vi "svfa_Process Frequency Response Subset.vi"(0 "Windowed signal [X]":waveform(dbl)={"t0"=timestamp(0 s since 1904-01-01), "dt"=1.953125e-05, "Y"=[]}, 1 "Windowed signal [Y]":waveform(dbl)={"t0"=timestamp(0 s since 1904-01-01), "dt"=1.953125e-05, "Y"=[]}, 2 "window (includes Force_Exp)":T9(ring), 3 "force/exp settings":T8={"force window [%]"=50.0, "exponential window [%]"=10.0} {"exponential window [%]" min=0.0 max=100.0 format="%.2f"; "force window [%]" min=0.0 max=100.0 format="%.2f"}, 4 "averaging parameters":T12={"averaging mode"=enum."No averaging", "weighting mode"=enum."Linear", "number of averages"=10, "linear mode"=enum."Auto restart"}, 5 "error in (no error)":errorcluster, 6 "Spectrum Settings":T10 {"stop frequency" format="%.2f"; "start frequency" format="%.2f"}, 7 "processing control":T7(ring), 9 "FRF mode":enum16{"H1", "H2", "H3"}(ring)) -> (12 "averages completed":dbl format="%.2f", 13 "processing control":T7(ring), 14 "complex frequency response":T11={"f0"=0.0, "df"=1.0, "complex spectrum"=[]} {"complex spectrum" format="%.2f"; "df" format="%.2f"; "f0" format="%.2f"}, 16 "Coherence":cluster{"f0":dbl, "df":dbl, "Spectrum":dbl[]} {"Spectrum" format="%.2f"; "df" format="%.2f"; "f0" format="%.2f"}, 17 "averaging done":bool, 18 "spectrum info":T1={"channel name"="", "description"="", "x-axis units"=0, "spectral info"={"spectrum type"=enum."Power [Magnitude^2]", "linear/dB"=enum."linear", "window"=0, "window size"=0, "FFT size"=0}, "engineering units"=1, "custom label"="", "dB reference [EU]"=0.0, "peak units"=enum."rms", "weighting filter"=0, "spectral density?"=FALSE, "unit label"="", "spectrum skewed?"=FALSE, "complimentary spectrum units"=enum."none"} {"x-axis units" items=["Time (s)"=0, "Frequency-CB (Hz)"=1, "Frequency-CPB (Hz)"=1248, "Frequency-Arbitrary (Hz)"=2357, "Quefrency (s)"=2, "Revolutions (rev)"=3, "Order"=4, "Speed (RPM)"=11, "Speed (rad/s)"=21, "Index"=65535]; "weighting filter" items=["Linear", "A-weighting", "B-weighting", "C-weighting", "ITU-R 468-4", "Dolby", "CCITT", "C-message", "Wb", "Wc", "Wd", "We", "Wf", "Wh", "Wj", "Wk", "Wm", "AES17 20 kHz lowpass", "AES17 40 kHz lowpass", "AES17 20 kHz highpass", "AES17 40 kHz highpass"]; "dB reference [EU]" format="%.2f"; "engineering units" items=["custom..."=0, "V"=1, "A"=21, "C"=30, "pC"=31, "s"=32, "-"=29, "Pa"=2, "N"=20, "g"=3, "m/s^2"=4, "m/s"=5, "m"=6, "mm/s"=12, "mm"=13, "micron/s"=14, "micron"=15, "in/s^2"=7, "in/s"=8, "in"=9, "mil/s"=10, "mil"=11, "rad/s^2"=16, "rad/s"=17, "rad"=18, "deg/s^2"=26, "deg/s"=27, "deg"=28, "RPM"=22, "cycle/s^2"=23, "Hz"=24, "cycle"=25, "strain"=19]; "spectral info"."window" items=["None "=0, "Hanning"=1, "Hamming"=2, "Blackman-Harris"=3, "Exact Blackman"=4, "Blackman"=5, "Flat Top"=6, "4 Term B-Harris "=7, "7 Term B-Harris"=8, "Low Sidelobe"=9, "Force - Exponential"=10, "Gaussian"=62]}, 19 "error out":errorcluster)   [LabVIEW 2017]
uses:
  <vilib>/addons/_NISVFA/_Shared subVIs/Controls/svc_Spectrum Info.ctl
  <vilib>/addons/_NISVFA/_Shared subVIs/Controls/svc_X-Axis Units.ctl
  <vilib>/addons/_NISVFA/_Shared subVIs/Controls/svc_Spectrum Type.ctl
  <vilib>/addons/_NISVFA/_Shared subVIs/Controls/svc_Engineering Units Text Ring.ctl
  <vilib>/addons/_NISVFA/_Shared subVIs/Controls/svc_Weighting Filter Text Ring.ctl
  <vilib>/addons/_NISVFA/_Shared subVIs/Controls/svc_Complimentary Spectrum Units.ctl
  <vilib>/addons/_NISVFA/_Shared subVIs/Windowing/svfa_Scaled Time Domain Window (1 Ch).vi
  <vilib>/addons/_NISVFA/_Shared subVIs/Windowing/svfa_Scaled Time Domain Window (Array).vi
  <vilib>/Analysis/4window.llb/Force Window.vi
  <vilib>/Analysis/4window.llb/Force Window (DBL).vi
  <vilib>/Analysis/4window.llb/Exponential Window.vi
  <vilib>/Analysis/4window.llb/Exponential Window (DBL).vi
  <vilib>/Utility/error.llb/Error Cluster From Error Code.vi
  <vilib>/Analysis/0measdsp.llb/Scaled Time Domain Window.vi
  <vilib>/Analysis/0measdsp.llb/Scaled Time Domain Window (DBL).vi
  <vilib>/addons/_NISVFA/_Spectrum Processing/subVIs/svfa_Spectrum Info Window to windowTd Type Def.vi
  <vilib>/addons/_NISVFA/_Shared subVIs/Common/svc_Window Parameters.vi
  <vilib>/addons/_NISVFA/_Shared subVIs/Common/svc_Get Window Info.vi
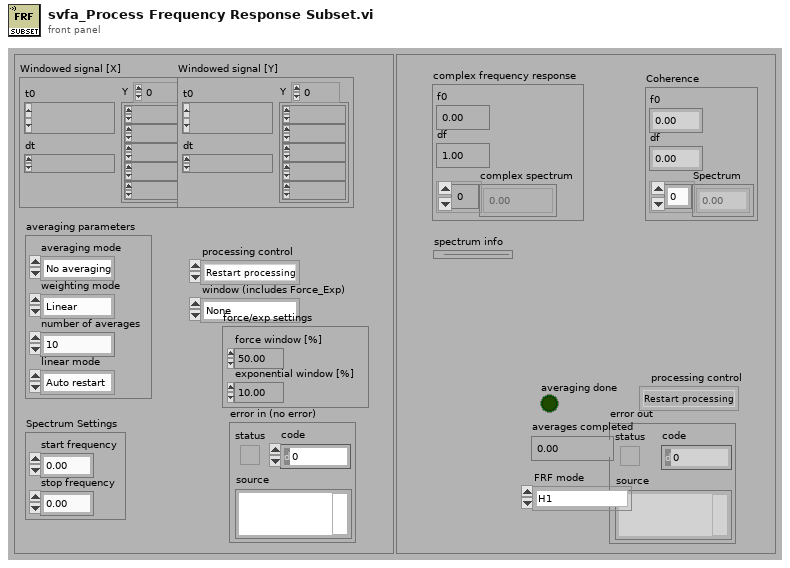
[diagram p1: front panel]
types:
  T1 = typedef "svc_Spectrum Info.ctl" = cluster{"channel name":string, "description":string, "x-axis units":T2, "spectral info":cluster{"spectrum type":T3, "linear/dB":enum16{"linear", "dB"}, "window":u16, "window size":i32, "FFT size":i32}, "engineering units":T4, "custom label":string, "dB reference [EU]":dbl, "peak units":enum16{"rms", "peak", "peak-peak"}, "weighting filter":T5, "spectral density?":bool, "unit label":string, "spectrum skewed?":bool, "complimentary spectrum units":T6}
  T2 = typedef "svc_X-Axis Units.ctl" = u16
  T3 = typedef "svc_Spectrum Type.ctl" = enum16{"FFT Spectrum [complex]", "Amplitude [Magnitude]", "Power [Magnitude^2]", "Cross Spectrum [complex]", "Frequency Response [Complex]"}
  T4 = typedef "svc_Engineering Units Text Ring.ctl" = u16
  T5 = typedef "svc_Weighting Filter Text Ring.ctl" = u16
  T6 = typedef "svc_Complimentary Spectrum Units.ctl" = enum16{"none", "radians", "degrees", "cycles", "imaginary"}
  T7 = enum16{"Restart processing", "Continue processing", "Skip processing"}
  T8 = cluster{"force window [%]":dbl, "exponential window [%]":dbl}
  T9 = enum16{"None ", "Hanning", "Hamming", "Blackman-Harris", "Exact Blackman", "Blackman", "Flat Top", "4 Term B-Harris ", "7 Term B-Harris", "Low Sidelobe", "Force - Exponential"}
  T10 = cluster{"start frequency":dbl, "stop frequency":dbl}
  T11 = cluster{"f0":dbl, "df":dbl, "complex spectrum":cdb[]}
  T12 = cluster{"averaging mode":enum16{"No averaging", "Vector averaging", "RMS averaging", "Peak hold"}, "weighting mode":enum16{"Linear", "Exponential"}, "number of averages":u32, "linear mode":enum16{"One shot", "Auto restart"}}
  T13 = typedef "svc_Window [Dual FFT].ctl" = u32
  T14 = cluster{"complex spectrum":cluster{"f0":dbl, "df":dbl, "complex spectrum":cdb[]}, "spectrum info":T1}
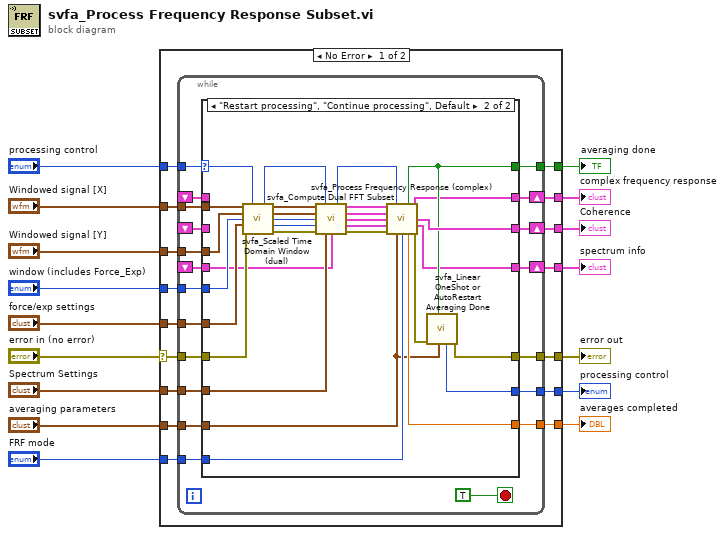
[diagram p0: block diagram]
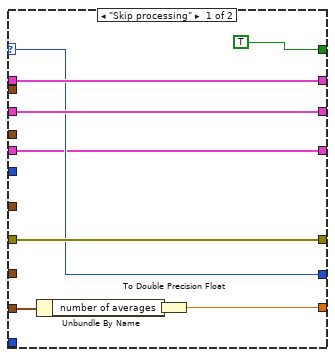
[diagram p2: hidden frame]
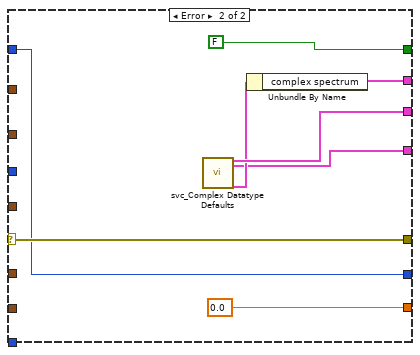
[diagram p3: hidden frame]
diagram:
  n1 = case shown="No Error" "error in (no error)" {
    selector: "error in (no error)" -> [w30 w99]
    tunnel: [w26 w99] -> w16
    tunnel: "averaging parameters" -> [w25 _]
    tunnel: "Windowed signal [X]" -> [w32 _]
    tunnel: "Windowed signal [Y]" -> [w31 _]
    tunnel: [w27 0.0 ("averages completed")] -> w11
    tunnel: [w18 w92] -> w10
    tunnel: [w19 w95] -> w9
    tunnel: "Spectrum Settings" -> [w29 _]
    tunnel: [w24 FALSE ("averaging done")] -> w7
    tunnel: "FRF mode" -> [w28 _]
    tunnel: "window (includes Force_Exp)" -> [w23 _]
    tunnel: "force/exp settings" -> [w22 _]
    tunnel: "processing control" -> [w21 w96]
    tunnel: [w20 w96] -> w2
    tunnel: [w17 w93] -> w1
    frame No Error {
      n2 = while {
        shift-left: _ -> [w35]
        shift-right: [w36] -> w19
        shift-left: _ -> [w37]
        shift-right: [w38] -> w18
        tunnel: [w40] -> w20
        tunnel: w21 -> [w39]
        tunnel: w22 -> [w45]
        tunnel: w23 -> [w46]
        tunnel: [w41] -> w24
        tunnel: w25 -> [w42]
        tunnel: [w50] -> w26
        tunnel: [w51] -> w27
        tunnel: w28 -> [w43]
        tunnel: w29 -> [w52]
        tunnel: w30 -> [w44]
        tunnel: w31 -> [w49]
        tunnel: w32 -> [w48]
        shift-right: [w34] -> w17
        shift-left: _ -> [w33]
        stop <- TRUE stop-if-true
        n3 = case shown="\"Restart processing\", \"Continue processing\", Default" w39 {
          selector: w39 -> [w57 w66]
          tunnel: w52 -> [_ w71]
          tunnel: [w54 w90] -> w51
          tunnel: [w58 w69] -> w50
          tunnel: [w60 w76] -> w38
          tunnel: [w59 w89] -> w36
          tunnel: w49 -> [_ w88]
          tunnel: w48 -> [_ w87]
          tunnel: w46 -> [_ w84]
          tunnel: w45 -> [_ w83]
          tunnel: w44 -> [w58 w81]
          tunnel: w43 -> [_ w79]
          tunnel: w42 -> [w56 w68]
          tunnel: [TRUE ("averaging done") w78] -> w41
          tunnel: [w57 w67] -> w40
          tunnel: w37 -> [w60 _]
          tunnel: w35 -> [w59 _]
          tunnel: [w53 w63] -> w34
          tunnel: w33 -> [w53 w62]
          frame "Skip processing" {
            n4 = Unbundle By Name(w56) -> ("number of averages"=w55:u32)
            n5 = To Double Precision Float(number=w55) -> (double precision float=w54:dbl)
          }
          frame "Restart processing", "Continue processing", Default {
            n6 = call <vilib>:"svfa_Scaled Time Domain Window (dual).vi"("Signal in [X]"=w87, "processing control"=w66, "Signal in [Y]"=w88, "window"=w84, "force/exp settings"=w83, "error in (no error)"=w81) -> ("dup processing control"=w65:T7, "Windowed signal [X]"=w86:waveform(dbl), "Windowed signal [Y]"=w85:waveform(dbl), "window"=w73:T13, "window size"=w72:i32, "error out"=w82:errorcluster)  [unwired: 3 in, 1 out]
            n7 = call <vilib>:"svfa_Compute Dual FFT Subset.vi"("Windowed signal [X]"=w86, "processing control"=w65, "Windowed signal [Y]"=w85, "window"=w73, "window size"=w72, "error in (no error)"=w82, "Spectrum Settings"=w71, "spectrum info in"=w62) -> ("dup processing control"=w64:T7, "X FFT spectrum [Vrms]"=w91:cluster{"f0":dbl, "df":dbl, "spectrum":cdb[]}, "spectrum info X"=w75:T1, "Y FFT spectrum [Vrms]"=w77:cluster{"f0":dbl, "df":dbl, "spectrum":cdb[]}, "spectrum info Y"=w74:T1, "error out"=w80:errorcluster)  [unwired: 2 in]
            n8 = call <vilib>:"svfa_Process Frequency Response (complex).vi"("X FFT spectrum [Vrms]"=w91, "processing control"=w64, "spectrum info X"=w75, "Y FFT spectrum [Vrms]"=w77, "spectrum info Y"=w74, "error in (no error)"=w80, "averaging parameters"=w68, "FRF mode"=w79) -> ("averaging done"=w78:bool, "complex spectrum"=w76:T11, "coherence"=w89:cluster{"f0":dbl, "df":dbl, "spectrum":dbl[]}, "spectrum info"=w63:T1, "averages completed"=w90:dbl, "error out"=w70:errorcluster)  [unwired: 2 in]
            n9 = call <vilib>:"svfa_Linear OneShot or AutoRestart Averaging Done.vi"("averaging parameters"=w68, "averaging done"=w78, "error in (no error)"=w70) -> ("error out"=w69:errorcluster, "processing control"=w67:T7)  [unwired: 7 in]
          }
        }
      }
    }
    frame Error {
      n10 = call <vilib>:"svc_Complex Datatype Defaults.vi"() -> ("empty spectrum"=w95:cluster{"f0":dbl, "df":dbl, "magnitude":dbl[]}, "dead spectrum info"=w93:T1, "complex spectrum"=w94:T14)  [unwired: 11 in, 6 out]
      n11 = Unbundle By Name(w94) -> ("complex spectrum"=w92:T11)
    }
  }
  "error out" <- w16
  "averages completed" <- w11
  "averaging done" <- w7
  "complex frequency response" <- w10
  "Coherence" <- w9
  "processing control" <- w2
  "spectrum info" <- w1
